vi "Feeder.vi"(11 "Feeder motor":bool) -> ()   [LabVIEW 2017]
uses:
  Robot Global Data.vi
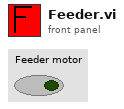
[diagram p1: front panel]
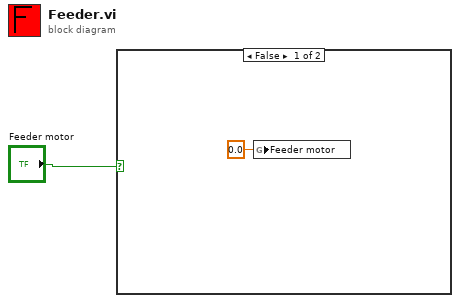
[diagram p0: block diagram]
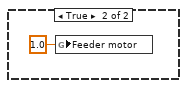
[diagram p2: hidden frame]
diagram:
  n1 = case shown="False" "Feeder motor" {
    frame False {
      n2 = global write "Robot Global Data.vi" "Feeder motor"(0.0 ("Feeder motor")) -> ()
    }
    frame True {
      n3 = global write "Robot Global Data.vi" "Feeder motor"(1.0 ("Feeder motor")) -> ()
    }
  }
